vi "Number_dbl to decimal string.vi"(11 "Number In":dbl) -> (3 "resulting string":string)   [LabVIEW 2021]
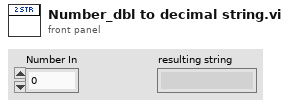
[diagram p1: front panel]
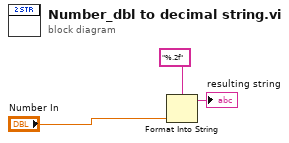
[diagram p0: block diagram]
diagram:
  n1 = Format Into String(format string="%.2f", "Number In") -> (resulting string=→"resulting string":string)  [unwired: 2 in, 1 out]
